vi "RCfilter.vi"() -> ()   [LabVIEW 2020]
panel:
  out "Phase":dbl
  out "Phi":dbl
  out "Cut off [f]":dbl=720.4841244540306
  in  "Cap":dbl=4.7e-08
  in  "Res":dbl=4700.0
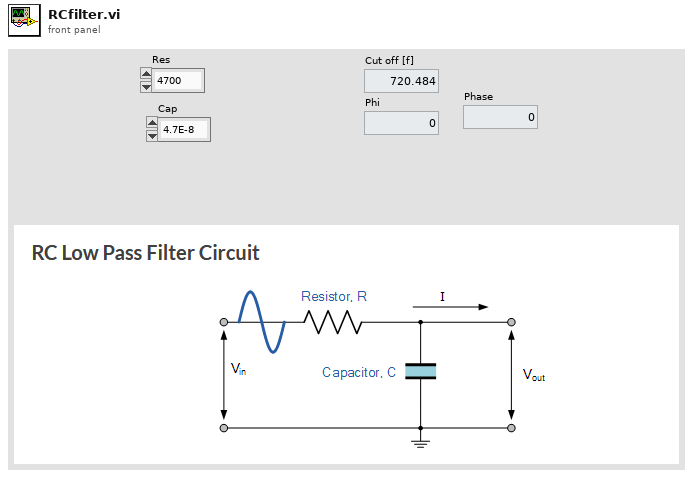
[diagram p1: front panel]
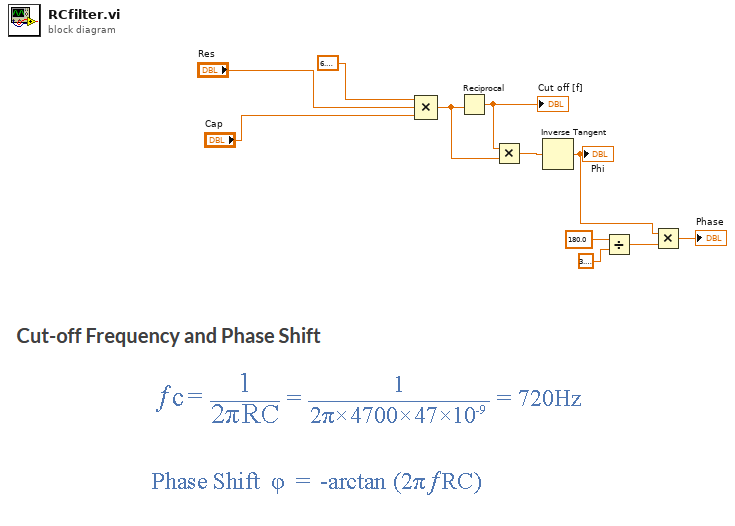
[diagram p0: block diagram]
diagram:
  n1 = Compound Arithmetic op=MULTIPLY(6.283185307179586, "Res", "Cap") -> (w7:dbl)
  n2 = Reciprocal(x=w7) -> (1/x=w8:dbl)
  "Cut off [f]" <- w8
  n3 = Multiply(x=w8, y=w7) -> (x*y=w6:dbl)
  n4 = Inverse Tangent(1:w6) -> (0:w2:dbl)
  "Phi" <- w2
  n5 = Divide(x=180.0, y=3.141592653589793) -> (x/y=w4:dbl)
  n6 = Multiply(x=w2, y=w4) -> (x*y=→"Phase":dbl)
